vi "Globals.vi"() -> ()   [LabVIEW 2020]
panel:
  out "Request_URL":string
  out "Body":string
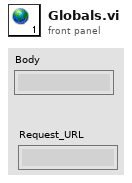
[diagram p1: front panel]
diagram:
